vi "Create ImageData Buffer.vi"(5 "Buffer Name":string, 7 "CircularBuffer.ImageData":refnum<class "CircularBuffer.ImageData.lvclass">, 8 "error in (no error)":errorcluster, 11 "BufferSize":i32=1) -> (0 "error out":errorcluster, 2 "Buffer name created":string, 3 "CircularBuffer.ImageData out":refnum<class "CircularBuffer.ImageData.lvclass">)   [LabVIEW 2015, in "CircularBuffer.ImageData.lvclass"]
uses:
  CircularBuffer.ImageData.lvclass
  CircularBuffer/types/type.ImageData/type.ImageData.lvclass
  CircularBuffer/CircularBuffer.lvclass
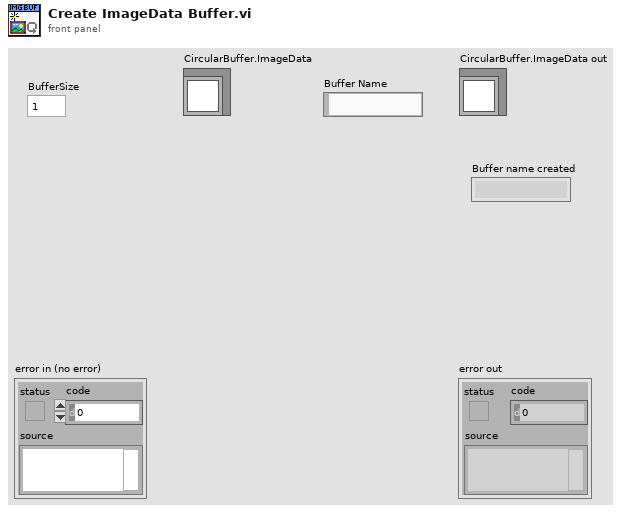
[diagram p1: front panel]
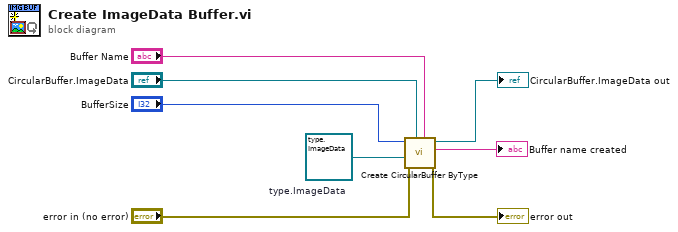
[diagram p0: block diagram]
diagram:
  w8 = refnum<class "type.ImageData.lvclass"> refnum  # type.ImageData
  n1 = call "Create CircularBuffer ByType.vi"("Buffer Name"="Buffer Name", "CircularBuffer in"="CircularBuffer.ImageData", "error in (no error)"="error in (no error)", "type"=w8, "BufferSize"="BufferSize") -> ("error out"=→"error out":errorcluster, "Buffer name created"=→"Buffer name created":string, "CircularBuffer out"=→"CircularBuffer.ImageData out":refnum<class "CircularBuffer.ImageData.lvclass">)  [unwired: 4 in]
